vi "FXPTriangleGen.vi"(10 "triangleInc":fxp<+/-,16,1>) -> (3 "triangle":fxp<+/-,32,4>)   [LabVIEW 2015, in "SPWM.lvlib"]
doc: "This VI generates the next point on a DDS generated sine wave.\n\nThe accumulator increments to calculate the next phase value in the waveform. By varying the accumulator increment you control the frequency of the sine wave.\n\nThe accumulator phase value is used to select a value from the sine wave reference waveform stored in the Lookup Table VI. The waveformcan be p[hase shifted by specifying a non-zero phase shift value which is added to the accumulator phase. The output from the LUT is scaled using the AO Amplitude value."
uses:
  SPWM.lvlib
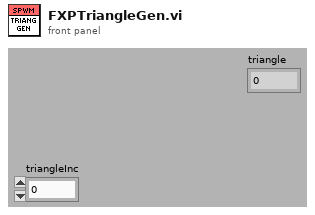
[diagram p1: front panel]
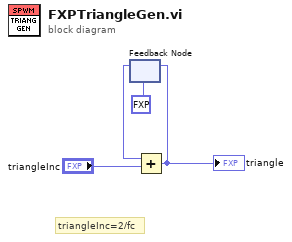
[diagram p0: block diagram]
diagram:
  # "triangleInc=2/fc"
  n1 = feedback #1(fxp<+/-,16,1> 0.0 ("triangle")) -> (w3:fxp<+/-,16,1>)
  n2 = Add(x=w3, y="triangleInc") -> (x+y=w1:fxp<+/-,16,1>)
  "triangle" <- w1
  n3 = feedback-in #1(w1) -> ()
